vi "hardware status globals.vi"() -> ()   [LabVIEW 2015]
uses:
  shutters status.ctl
  new-h-nu-ixon/Laser type.ctt
  new-h-nu-ixon/Emission filters.ctl
panel:
  in  "Emission filter status":T1
  out "Camera status":bool
  in  "Shutters Status":T2=[{"Laser"=enum."Blue 488 nm", "Status"=FALSE}, {"Laser"=enum."Green 532 nm", "Status"=FALSE}, {"Laser"=enum."Red 633 nm", "Status"=FALSE}, {"Laser"=enum."IR 780", "Status"=FALSE}]
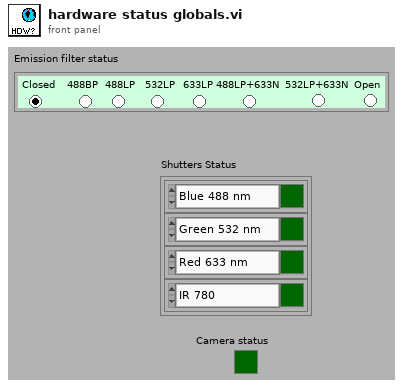
[diagram p1: front panel]
types:
  T1 = typedef "Emission filters.ctl" = enum32{" Closed ", " 488BP ", "488LP", "  532LP ", "633LP", "488LP+633N", "532LP+633N", "Open"}
  T2 = typedef "shutters status.ctl" = cluster{"Laser":T3, "Status":bool}[]
  T3 = typedef "Laser type.ctt" = enum16{"Blue 488 nm", "Green 532 nm", "Red 633 nm", "IR 780"}
diagram:
